vi "Call ADB non blocking.vi"(3 "error in":errorcluster, 4 "adb sub-command":string, 5 "adb location":string) -> (0 "error out":errorcluster)   [LabVIEW 2016]
doc: "Calls the ADB command line utility at \"adb location\" or default /usr/bin/adb with \"adb sub-command\". The \"adb sub-command\" should include all arguements formatted as appropriate for a command line utility."
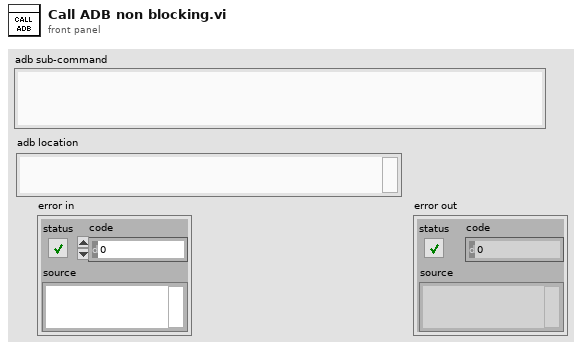
[diagram p1: front panel]
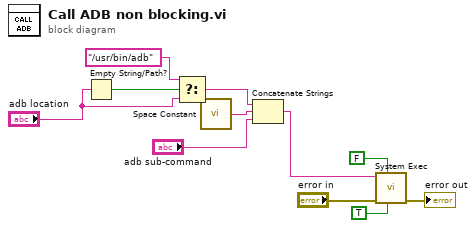
[diagram p0: block diagram]
diagram:
  n1 = Empty String/Path?(string/path="adb location") -> (empty?=w10:bool)
  n2 = Select(t="/usr/bin/adb" ("name or relative path"), s=w10, f="adb location") -> (s? t:f=w3:string)
  n3 = call <vilib>:"Space Constant.vi"() -> ("String"=w5:string)
  n4 = Concatenate Strings(w3, w5, "adb sub-command") -> (w2:string)
  n5 = call <vilib>:"System Exec.vi"("run minimized? (F)"=TRUE, "wait until completion? (T)"=FALSE, "error in (no error)"="error in", "command line"=w2) -> ("error out"=→"error out":errorcluster)  [unwired: 4 in, 3 out]
